vi "Configure Max Output Voltage.vi"(0 "VISA resource name":refnum<visa-resource-name>, 2 "Communication Address (0)":i16 max=254 format="%x", 7 "Maximum Output Voltage (18)":dbl=18.0 min=0.0 max=72.0 format="%#.2g", 11 "error in (no error)":errorcluster) -> (4 "VISA resource name out":refnum<visa-resource-name>, 15 "error out":errorcluster)   [LabVIEW 2015, in "BK Precision 178XB Series.lvlib"]
doc: "This VI configures the maximum output voltage. This value acts as an overvoltage protection, thus limiting the voltage any device is allowed to draw from the supply. No voltage values will exceed this configured value from the supply. If a voltage higher than this set value is being drawn from a device, the supply will not allow it and limit voltage to this value."
uses:
  <instrlib>/BK Precision 178XB Series/BK Precision 178XB Series.lvlib
panel:
  # "(c) 2009 B&K PRECISION CORPORATION.  ALL RIGHTS RESERVED."
  # "Note:  Maximum Output Voltage limits to 18 V by default based on model 1785B maximum rated voltage.  For 1786B and 1788models, maximum can be 32 V.  For 1787B, maximum can be up to 72 V."
  # "V"
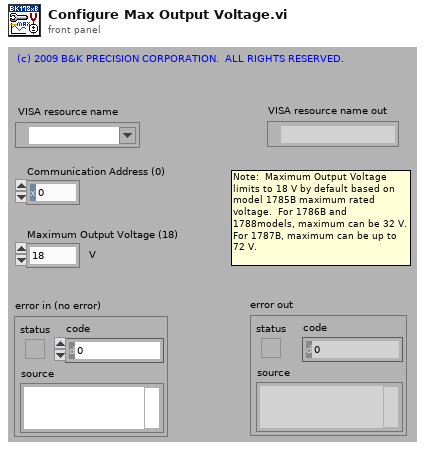
[diagram p1: front panel]
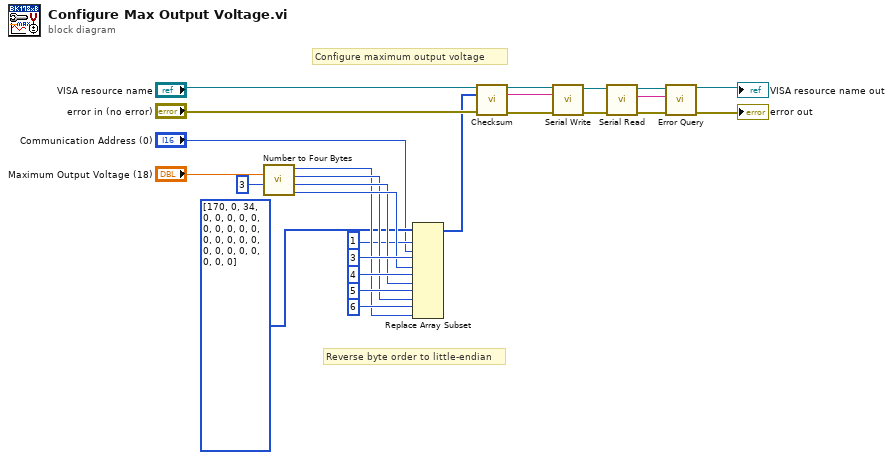
[diagram p0: block diagram]
diagram:
  # "Reverse byte order to little-endian"
  # "Configure maximum output voltage"
  n1 = call <instrlib>:"Number to Four Bytes.vi"("Fractional Precision (3)"=3 ("index"), "Input Value (0)"="Maximum Output Voltage (18)") -> ("Byte 4"=w21:i32, "Byte 3"=w20:i32, "Byte 2"=w19:i32, "Byte 1"=w18:i32)  [unwired: 6 in]
  n2 = Replace Array Subset(array=i16[] [170, 0, 34, 0, 0, 0, 0, 0, 0, 0, 0, 0, 0, 0, 0, 0, 0, 0, 0, 0, 0, 0, 0, 0, 0, 0], new element #1="Communication Address (0)", index #1=1, new element #2=w21, index #2=3 ("index"), new element #3=w20, index #3=4 ("index"), new element #4=w19, index #4=5 ("index"), new element #5=w18, index #5=6 ("index")) -> (w8:i16[])
  n3 = call <instrlib>:"Checksum.vi"("VISA resource name"="VISA resource name", "Command Frame Array"=w8, "error in (no error)"="error in (no error)") -> ("VISA resource name out"=w7:refnum<visa-resource-name>, "Output String"=w5:string, "error out"=w6:errorcluster)  [unwired: 8 in, 2 out]
  n4 = call <instrlib>:"Serial Write.vi"("error in (no error)"=w6, "Input Command Frame"=w5, "VISA resource name"=w7) -> ("error out"=w17:errorcluster, "VISA resource name out"=w16:refnum<visa-resource-name>)  [unwired: 6 in, 1 out]
  n5 = call <instrlib>:"Serial Read.vi"("error in (no error)"=w17, "VISA resource name"=w16) -> ("error out"=w13:errorcluster, "Read Buffer"=w11:string, "VISA resource name out"=w12:refnum<visa-resource-name>)  [unwired: 7 in]
  n6 = call <instrlib>:"Error Query.vi"("VISA resource name"=w12, "Input Read Buffer 1"=w11, "error in (no error)"=w13) -> ("VISA resource name out"=→"VISA resource name out":refnum<visa-resource-name>, "error out"=→"error out":errorcluster)  [unwired: 7 in, 4 out]
